vi "guassian_fit_test.vi"() -> ()   [LabVIEW 2014]
panel:
  in  "Y Values":dbl[](array[numeric])=[0.0, 0.0, 0.0, 0.0, 0.0, 1.0, 2.0, 5.0, 15.0, 48.0, 51.0, 19.0, 7.0, 3.0, 1.0, 0.0, 0.0, 0.0, 0.0]
  out "offset":dbl
  out "FWHM":dbl
  out "Spread":dbl
  out "Center":dbl
  out "Amplitude":dbl
  out "XY Graph":cluster{dbl[], dbl[]}[](graph)
  in  "X Values":dbl[](array[numeric])=[1.0, 2.0, 3.0, 4.0, 5.0, 6.0, 7.0, 8.0, 9.0, 10.0, 11.0, 12.0, 13.0, 14.0, 15.0, 16.0, 17.0, 18.0, 19.0]
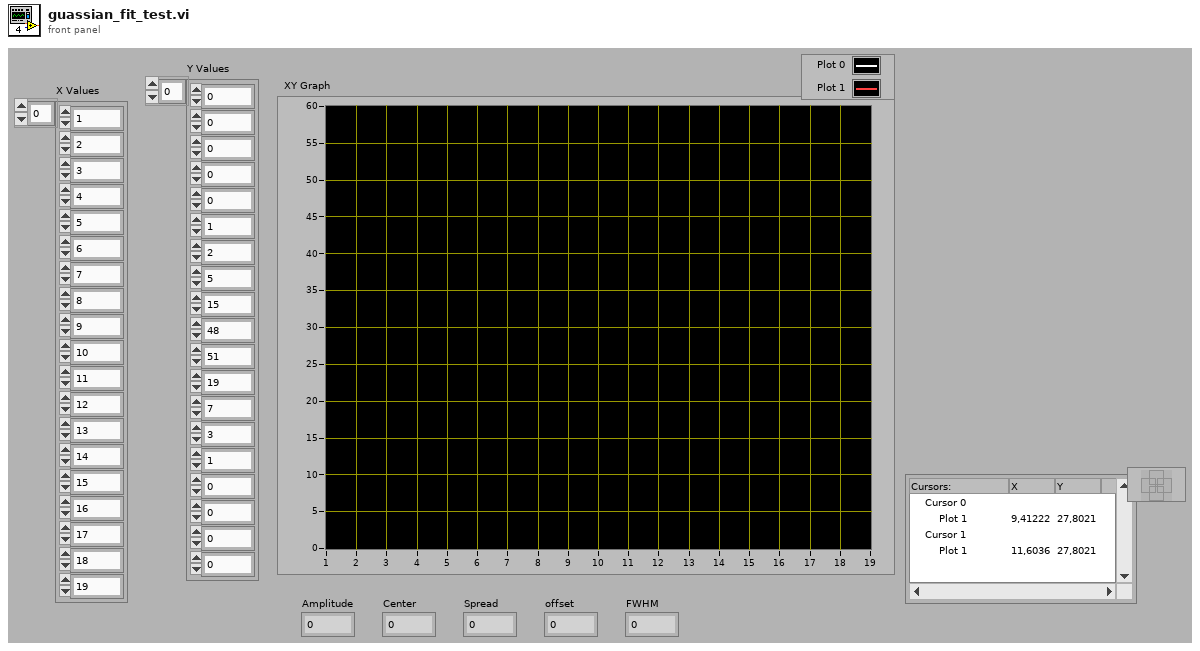
[diagram p1: front panel]
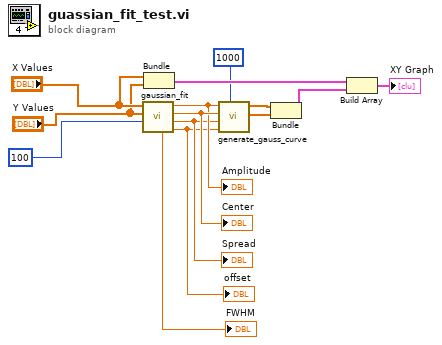
[diagram p0: block diagram]
diagram:
  n1 = call "gaussian_fit.vi"("Max Itterations"=100, "Y Values"="Y Values", "X Values"="X Values") -> ("offset"=w3:dbl, "Spread (st dev)"=w4:dbl, "Center"=w7:dbl, "Amplitude"=w5:dbl, "FWHM"=→"FWHM":dbl)  [unwired: 1 in, 1 out]
  "Amplitude" <- w5
  "Center" <- w7
  "Spread" <- w4
  "offset" <- w3
  n2 = Bundle("X Values"="X Values", "Y Values"="Y Values") -> (w13:cluster{"X Values":dbl[], "Y Values":dbl[]})  [unwired: 1 in]
  n3 = call "generate_gauss_curve.vi"("num points"=1000, "offset"=w3, "Spread"=w4, "Center"=w7, "Amplitude"=w5) -> ("Y Values"=w9:dbl[], "X Values"=w8:dbl[])  [unwired: 3 in]
  n4 = Bundle("X Values"=w8, "Y Values"=w9) -> (w12:cluster{"X Values":dbl[], "Y Values":dbl[]})  [unwired: 1 in]
  n5 = Build Array(w13, w12) -> (→"XY Graph":cluster{"X Values":dbl[], "Y Values":dbl[]}[])
